vi "MFLI_set_frequency -- V1.vi"(4 "Oscillator (0)":u16, 8 "Error In":errorcluster, 9 "timeconstant (s)":dbl=0.006, 10 "Freq in (Hz)":dbl=40000.0 format="%#_13g", 11 "Handle In":T1 {"Handle" format="0x%08x"; "Conn" format="0x%08x"}) -> (0 "Error Out":errorcluster, 1 "z out (V)":cdb, 2 "Freq out (Hz)":dbl=40000.0 format="%#_13g", 3 "Handle Out":T1 {"Handle" format="0x%08x"; "Conn" format="0x%08x"})   [LabVIEW 2017]
uses:
  <instrlib>/Zurich Instruments LabOne/Public/ziTypeHandle.ctl
  <instrlib>/Zurich Instruments LabOne/Zurich Instruments LabOne.lvlib
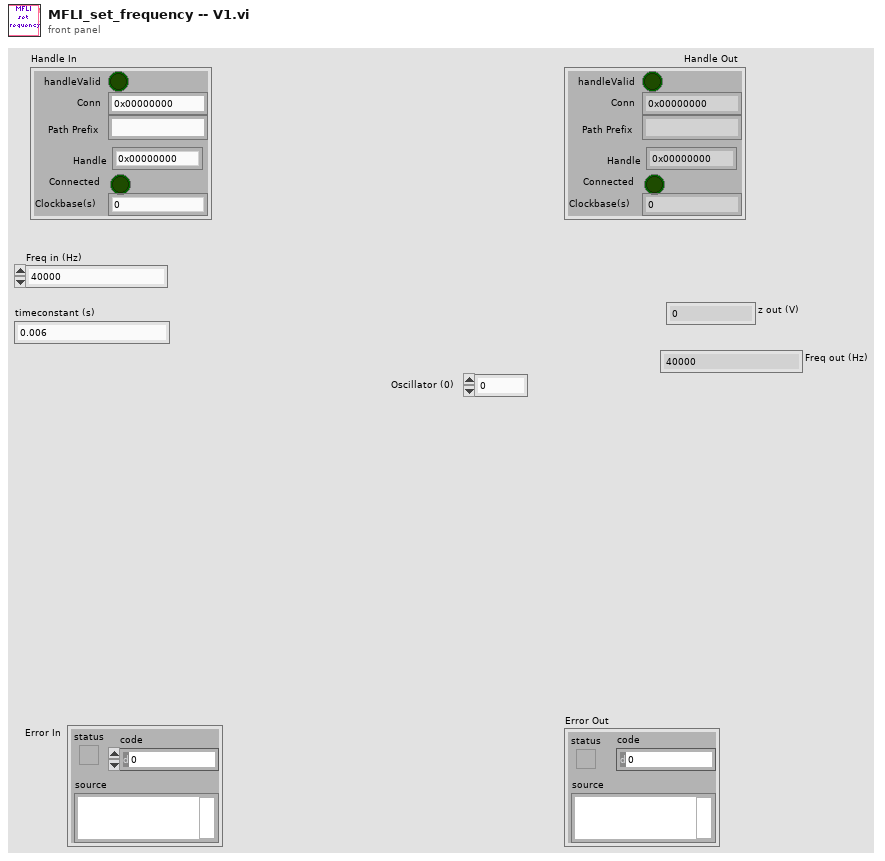
[diagram p1: front panel]
types:
  T1 = typedef "Zurich Instruments LabOne.lvlib/ziTypeHandle.ctl" = cluster{"handleValid":bool, "Conn":u64, "Path Prefix":string, "Handle":u64, "Connected":bool, "Clockbase(s)":dbl}
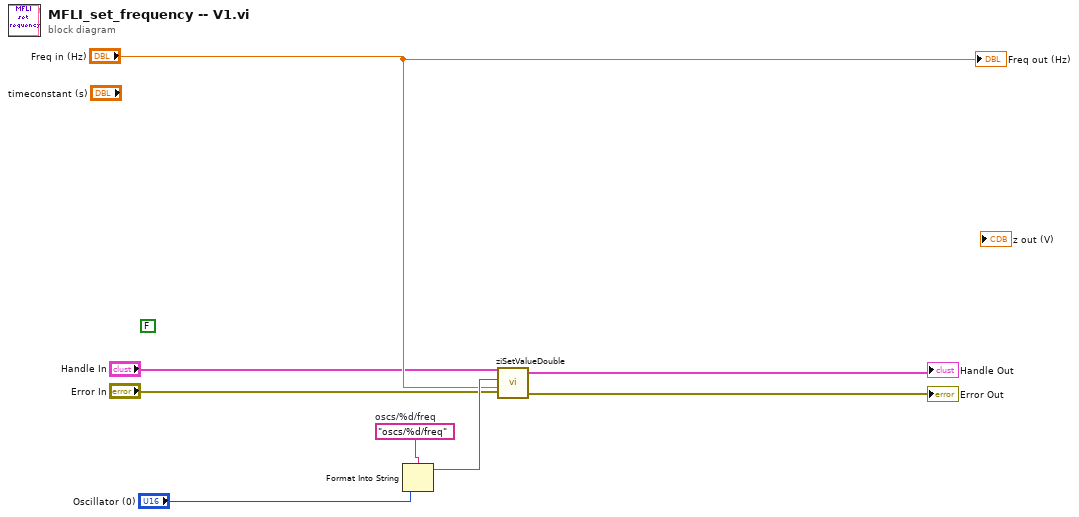
[diagram p0: block diagram]
diagram:
  (unwired) FALSE
  w8 = "oscs/%d/freq"  # oscs/%d/freq
  n1 = Format Into String(format string=w8, "Oscillator (0)") -> (resulting string=w7:string)  [unwired: 2 in, 1 out]
  n2 = call <instrlib>:"ziSetValueDouble.vi"("Error In"="Error In", "Value"="Freq in (Hz)", "Path"=w7, "Handle In"="Handle In") -> ("Error Out"=→"Error Out":errorcluster, "Handle Out"=→"Handle Out":T1)  [unwired: 1 in]
  "Freq out (Hz)" <- "Freq in (Hz)"
